vi "DFT_1024.vi"(10 "X":dbl[](array[numeric]), 11 "WaveformGraph in":refnum<vi>) -> (3 "Array":dbl[](array[numeric]))   [LabVIEW 2020]
uses:
  <vilib>/Analysis/2dsp.llb/Real FFT.vi
  <vilib>/Analysis/NI_AALPro.lvlib
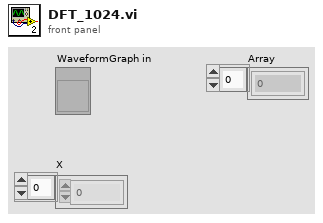
[diagram p1: front panel]
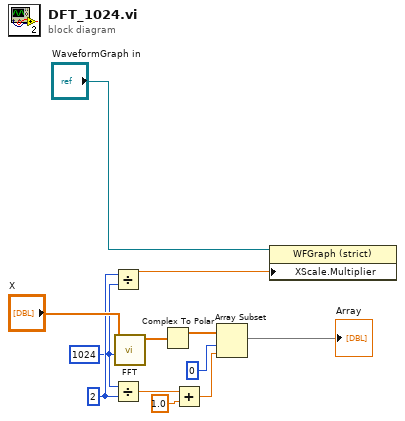
[diagram p0: block diagram]
diagram:
  w4 = 2 ("x")
  w3 = 1024 ("FFT size")
  n1 = Divide(x=w4, y=w3) -> (x/y=w2:dbl)
  n2 = Divide(x=w3, y=w4) -> (x/y=w7:dbl)
  n3 = call-poly <vilib>:"FFT.vi"("FFT size"=w3, "X"="X") -> ("FFT {X}"=w10:cdb[])  [unwired: 8 in, 1 out]
  n4 = Complex To Polar(r * e^(i*theta)=w10) -> (r=w9:dbl[])  [unwired: 1 out]
  n5 = Add(x=w7, y=1.0) -> (x+y=w5:dbl)
  n6 = Array Subset(array=w9, index=0, length=w5) -> (→"Array":dbl[])
  n7 = property on="Property Node" class="WFGraph (strict)"(reference="WaveformGraph in", "XScale.Multiplier"=w2) -> ()  [unwired: 1 in, 2 out]
